vi "Child Transport.vi"(6 "Unified Actor Alias":string, 7 "Actor in":refnum<class "Actor.lvclass">) -> (0 "Error out":errorcluster, 2 "Transport":refnum<user-event>)   [LabVIEW 2020, in "jettl.lvlib" / "Read Unified Actor.lvlib"]
uses:
  Read Unified Actor.lvlib
  Actor Specific/Actor Specific.lvlib
  Actor Specific/Find Child Attributes.vi
  Actor/Actor.lvclass
  Msg Input/Msg Input.lvclass
  Msg Output/Msg Output.lvclass
  Msg/Msg.lvclass
  Unified Actor Relation.ctl
  jettl.lvlib
  Teller.ctl
  Msg.ctl
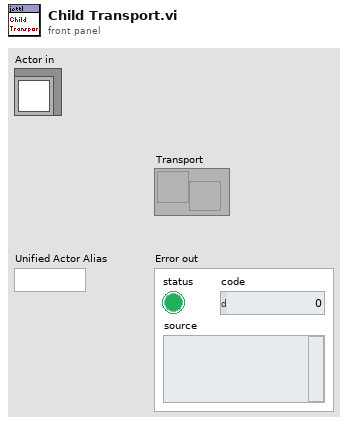
[diagram p1: front panel]
types:
  T1 = typedef "jettl.lvlib/Unified Actor.ctl" = cluster{"Msgs":T2, "Leaf":bool, "Edge Actors":refnum<class "Actor.lvclass">[], "Core Actors":refnum<class "Actor.lvclass">[], "Root":bool, "Alias":string, "DVR UID":i32, "Transport":refnum<user-event>, "Address":refnum<event-registration>, "This VI":refnum<vi>}
  T2 = typedef "jettl.lvlib/Msgs.ctl" = cluster{"Inbound":T3, "Outbound":T3, "Implemented":T3, "Tell Init":T3, "Tell Init Self":T3, "Tell Init Parent":T3, "Tell Init Child":T3, "Tell Forward":T3, "Tell Forward Self":T3, "Tell Forward Parent":T3, "Tell Forward Child":T3}
  T3 = typedef "jettl.lvlib/Msg Set.ctl" = set{refnum<class "Msg.lvclass">}
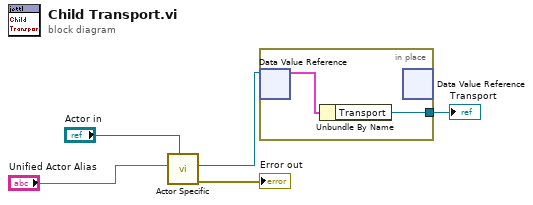
[diagram p0: block diagram]
diagram:
  n1 = call-poly "Actor Specific.vi"("Actor in"="Actor in", "Unified Actor Alias"="Unified Actor Alias") -> ("Error out"=→"Error out":errorcluster, "Child Unified Actor DVR"=w3:refnum<data-value>)  [unwired: 8 in]
  n2 = in-place {
    in-place-border: [w6] -> w1
    n3 = in-place-dvr #1(w3) -> (w7:T1)  [unwired: 1 out]
    n4 = Unbundle By Name(w7) -> ("Transport"=w6:refnum<user-event>)
    n5 = in-place-dvr #1() -> ()  [unwired: 1 in, 2 out]
  }
  "Transport" <- w1
